vi "clockCounter.vi"(3 "clock_divider_x":i16) -> (0 "Counter":i16, 1 "Clock":bool)   [LabVIEW 2016]
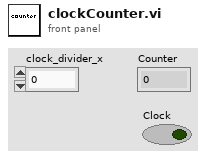
[diagram p1: front panel]
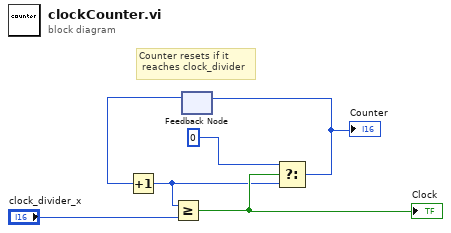
[diagram p0: block diagram]
diagram:
  # "Counter resets if it\n reaches clock_divider"
  n1 = feedback #1() -> (w4:u64)  [unwired: 1 in]
  n2 = Increment(x=w4) -> (x+1=w2:u64)
  n3 = Greater Or Equal?(x=w2, y="clock_divider_x") -> (x >= y?=w6:bool)
  "Clock" <- w6
  n4 = Select(t=u64 0, s=w6, f=w2) -> (s? t:f=w1:u64)
  "Counter" <- w1
  n5 = feedback-in #1(w1) -> ()
